vi "全局 水样时间.vi"() -> ()   [LabVIEW 2016, in "数据传输系统.lvlib"]
panel:
  in  "剖面多参数数据时间":string
  in  "水样数据索引":T1
  in  "选择发送的参数":string
  in  "小时数据时间":string
  in  "时间":string
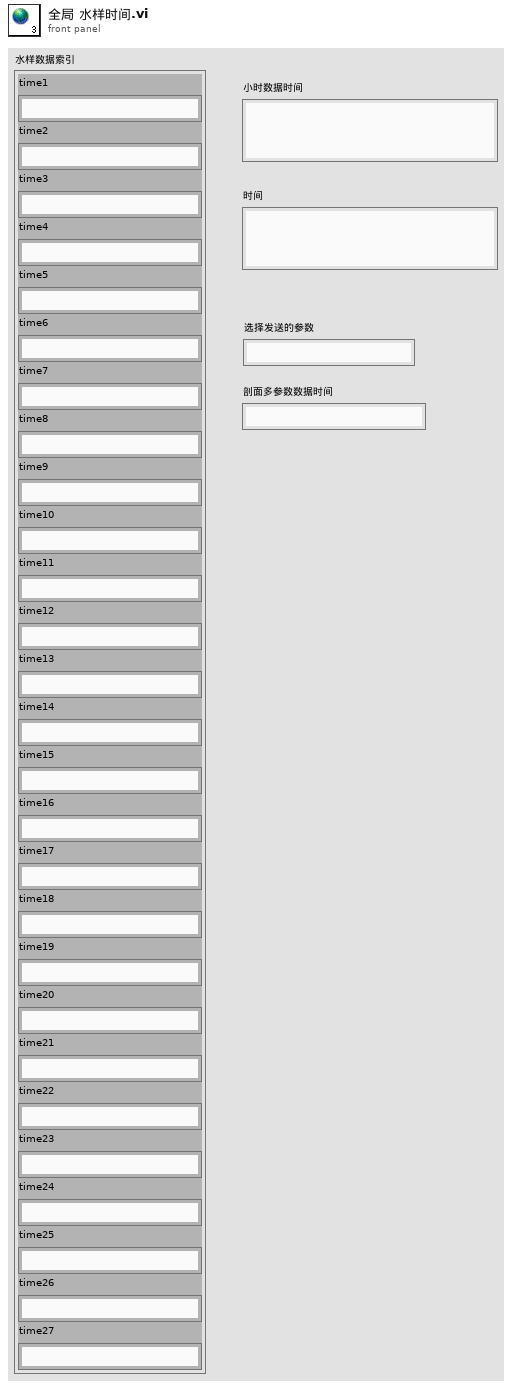
[diagram p1: front panel]
types:
  T1 = cluster{"time1":string, "time2":string, "time3":string, "time4":string, "time5":string, "time6":string, "time7":string, "time8":string, "time9":string, "time10":string, "time11":string, "time12":string, "time13":string, "time14":string, "time15":string, "time16":string, "time17":string, "time18":string, "time19":string, "time20":string, "time21":string, "time22":string, "time23":string, "time24":string, "time25":string, "time26":string, "time27":string}
diagram:
